vi "OP600ZP_FDT_V2.vi"(8 "errin":errorcluster, 9 "Tusine":dbl) -> (0 "errout":errorcluster, 2 "Log":string, 3 "is OK?":bool, 4 "ToBDD":T1)   [LabVIEW 2020]
uses:
  <userlib>/PCAN Basic/Controls/Channel.ctl
  VG/Ubatt.vi
  VG/PackType.vi
  VG/IS30%.vi
  OP600ZP_VGConf.vi
  <userlib>/PCAN Basic/PCANBasic.lvlib
panel:
  out "PASS/FAIL?":string
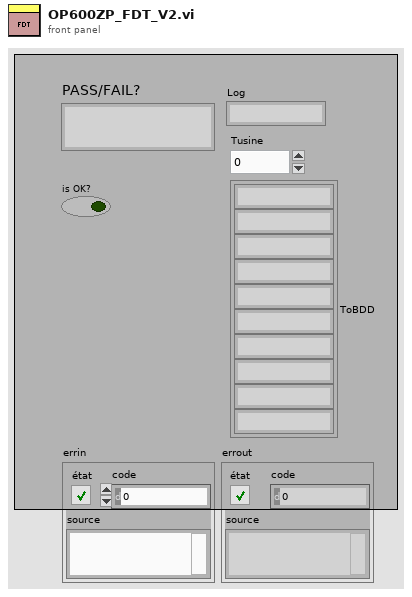
[diagram p1: front panel]
types:
  T1 = cluster{string, string, string, string, string, string, string, string, string, string}
  T2 = typedef "PCANBasic.lvlib/Channel.ctl" = enum16{"PCAN_NONEBUS", "not used1", "not used2", "not used3", "not used4", "not used5", "not used6", "not used7", "not used8", "not used9", "not used10", "not used11", "not used12", "not used13", "not used14", "not used15", "not used16", "not used17", "not used18", "not used19", "not used20", "not used21", "not used22", "not used23", "not used24", "not used25", "not used26", "not used27", "not used28", "not used29", "not used30", "not used31", "not used32", "PCAN_ISABUS1", "PCAN_ISABUS2", "PCAN_ISABUS3", "PCAN_ISABUS4", "PCAN_ISABUS5", "PCAN_ISABUS6", "PCAN_ISABUS7", "PCAN_ISABUS8", "not used41", "not used42", "not used43", "not used44", "not used45", "not used46", "not used47", "not used48", "PCAN_DNGBUS1", "not used50", "not used51", "not used52", "not used53", "not used54", "not used55", "not used56", "not used57", "not used58", "not used59", "not used60", "not used61", "not used62", "not used63", "not used64", "PCAN_PCIBUS1", "PCAN_PCIBUS2", "PCAN_PCIBUS3", "PCAN_PCIBUS4", "PCAN_PCIBUS5", "PCAN_PCIBUS6", "PCAN_PCIBUS7", "PCAN_PCIBUS8", "not used73", "not used74", "not used75", "not used76", "not used77", "not used78", "not used79", "not used80", "PCAN_USBBUS1", "PCAN_USBBUS2", "PCAN_USBBUS3", "PCAN_USBBUS4", "PCAN_USBBUS5", "PCAN_USBBUS6", "PCAN_USBBUS7", "PCAN_USBBUS8", "Not used89", "Not used90", "Not used91", "Not used92", "Not used93", "Not used94", "Not used95", "Not used96", "PCAN_PCCBUS1", "PCAN_PCCBUS2"}
  T3 = cluster{"F400 Battery Charge Type":string, "F400 Battery State Request":string, "F400 Ext Insulation Test Control":string, "F400 Int Insulation Test Control":string, "F400 Vehicle Speed":i32, "F400 Ambiant Temperature":i32, "F400 Charger Available Power":i32, "F400 Count":i32, "F106 Keep Active request":string, "F106 Battery State":string, "F106 Operating Status":string, "F106 Battery SOC":dbl, "F106 Battery SOH":dbl, "F106 Ext Insulation Test Status":string, "F106 Int Insulation Test Status":string, "F106 Power Distribution Status":string, "F106 Power Switch Off Delay":i32, "F106 Power Switch Off Request":string, "F106 Count":i32, "F101 Battery Voltage":u32, "F101 Battery Current":dbl, "F101 Max Charge Current":u32, "F101 Max Discharge Current":u32, "F101 Max Discharge Current Temp Limit":string, "F101 Max Discharge Current SOC Limit":string, "F101 Max Charge Current Temp Limit":string, "F101 Max Charge Current SOC Limit":string, "F101 Deliverable Energy":dbl, "F101 Count":u32, "F102 Cell Average Voltage":u32, "F102 Cell Min Voltage":u32, "F102 Cell Max Voltage":u32, "F103 Cell Average Temp":i32, "F103 Cell Min Temp":i32, "F102 Count":u32, "F103 SumOfInternalResistanceT":i32, "F100 Charge Voltage Setpoint":i32, "F100 Charge Current Setpoint":dbl, "F100 Equilization Status":bool, "F100 Charge Competed":bool, "F100 Count":i32, "F107 Outlet Water Temp Request":i32, "F107 Outlet Water Temp Status":i32, "F107 Flow Rate Request":i32, "F107 Inlet Water Temp":i32, "F107 Ambiant Temperature 2":i32, "F105 Max Power Charge Continuous":i32, "F105 Max Power Charge Long Prediction":i32, "F105 Max Power Charge Short Prediction":i32, "F105 Max Current Charge Continuous":i32, "F105 Max Current Charge Short Prediction":i32, "F105 Count ":i32, "F104 Max Power Discharge Continuous":i32, "F104 Max Power Discharge Long Prediction":i32, "F104 Max Power Discharge Short Prediction":i32, "F104 Max Current Discharge Continuous":i32, "F104 Max Current Discharge Short Prediction":i32, "F104 Count ":i32, "F103 Count":i32, "F103 Cell Max Temp":i32, "F103 Max Current Discharge Long Prediction":i32, "F103 Max Current Charge Long Prediction":i32, "F107 Count":i32, "F103 OCV":i32, "F109 DTC":i32}
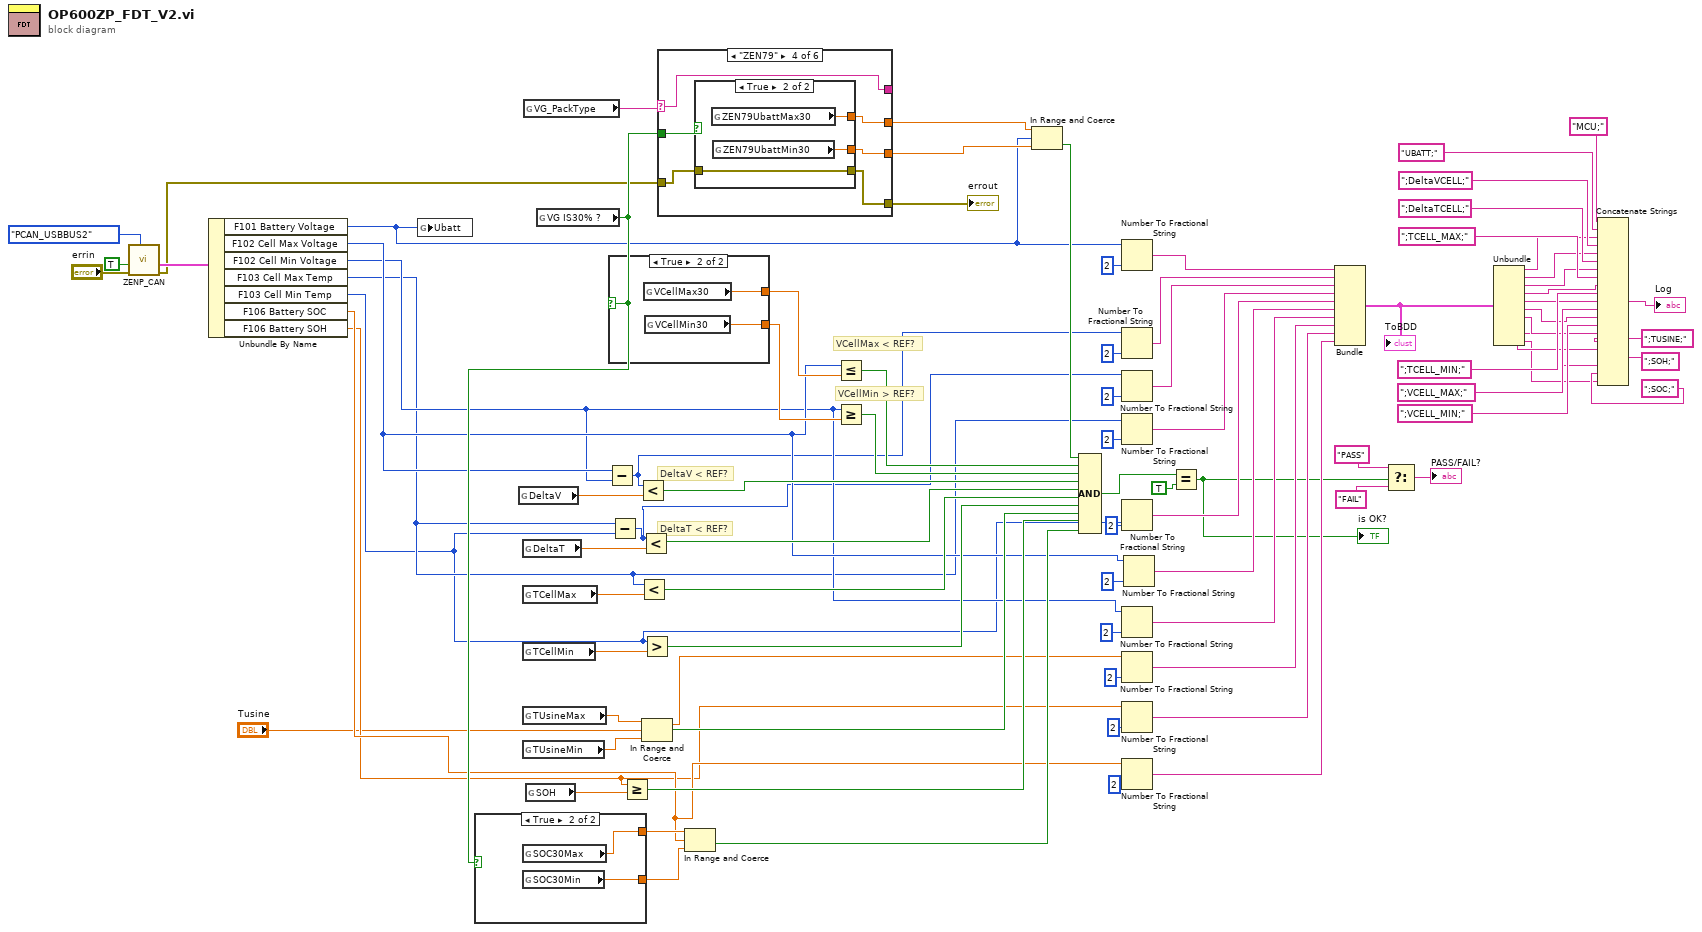
[diagram p0: block diagram]
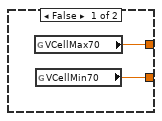
[diagram p2: hidden frame]
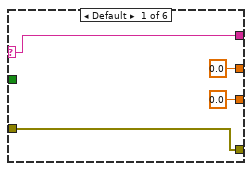
[diagram p3: hidden frame]
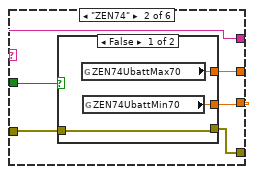
[diagram p4: hidden frame]
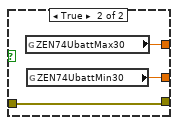
[diagram p5: hidden frame]
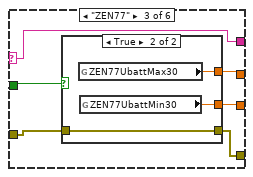
[diagram p6: hidden frame]
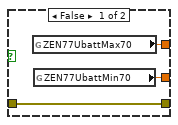
[diagram p7: hidden frame]
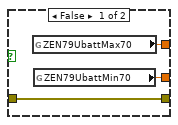
[diagram p8: hidden frame]
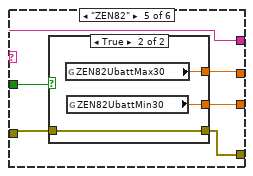
[diagram p9: hidden frame]
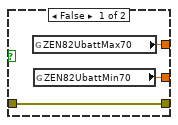
[diagram p10: hidden frame]
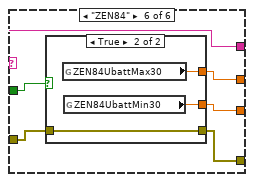
[diagram p11: hidden frame]
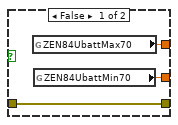
[diagram p12: hidden frame]
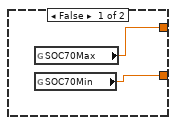
[diagram p13: hidden frame]
diagram:
  # "DeltaT < REF?"
  # "DeltaV < REF?"
  # "VCellMin > REF?"
  # "VCellMax < REF?"
  n1 = call <userlib>:"ZENP_CAN.vi"("Channel No Init"=Channel."PCAN_USBBUS2" ("Channel"), "errin"="errin", "Init?"=TRUE) -> ("errout"=w7:errorcluster, "data out"=w16:T3)  [unwired: 5 in, 1 out]
  n2 = Unbundle By Name(w16) -> ("F101 Battery Voltage"=w14:u32, "F102 Cell Max Voltage"=w13:u32, "F102 Cell Min Voltage"=w12:u32, "F103 Cell Max Temp"=w11:i32, "F103 Cell Min Temp"=w10:i32, "F106 Battery SOC"=w9:dbl, "F106 Battery SOH"=w8:dbl)
  n3 = global write "Ubatt.vi" "Ubatt"(w14) -> ()
  n4 = global read "OP600ZP_VGConf.vi" "DeltaV"() -> (w77:dbl)
  n5 = global read "OP600ZP_VGConf.vi" "DeltaT"() -> (w76:dbl)
  n6 = global read "OP600ZP_VGConf.vi" "TCellMax"() -> (w69:dbl)
  n7 = global read "OP600ZP_VGConf.vi" "TCellMin"() -> (w70:dbl)
  n8 = global read "OP600ZP_VGConf.vi" "TUsineMax"() -> (w64:dbl)
  n9 = global read "OP600ZP_VGConf.vi" "TUsineMin"() -> (w63:dbl)
  n10 = global read "PackType.vi" "VG_PackType"() -> (w91:string)
  n11 = global read "OP600ZP_VGConf.vi" "SOH"() -> (w29:dbl)
  n12 = global read "IS30%.vi" "VG IS30% ?"() -> (w32:bool)
  n13 = case shown="True" w32 {
    tunnel: [w93 w95] -> w31
    tunnel: [w92 w94] -> w30
    frame False {
      n14 = global read "OP600ZP_VGConf.vi" "SOC70Max"() -> (w93:dbl)
      n15 = global read "OP600ZP_VGConf.vi" "SOC70Min"() -> (w92:dbl)
    }
    frame True {
      n16 = global read "OP600ZP_VGConf.vi" "SOC30Max"() -> (w95:dbl)
      n17 = global read "OP600ZP_VGConf.vi" "SOC30Min"() -> (w94:dbl)
    }
  }
  n18 = Subtract(x=w13, y=w12) -> (x-y=w5:u32)
  n19 = case shown="True" w32 {
    tunnel: [w97 w99] -> w19
    tunnel: [w96 w98] -> w66
    frame False {
      n20 = global read "OP600ZP_VGConf.vi" "VCellMax70"() -> (w97:dbl)
      n21 = global read "OP600ZP_VGConf.vi" "VCellMin70"() -> (w96:dbl)
    }
    frame True {
      n22 = global read "OP600ZP_VGConf.vi" "VCellMax30"() -> (w99:dbl)
      n23 = global read "OP600ZP_VGConf.vi" "VCellMin30"() -> (w98:dbl)
    }
  }
  n24 = Subtract(x=w11, y=w10) -> (x-y=w4:i32)
  n25 = Greater Or Equal?(x=w8, y=w29) -> (x >= y?=w28:bool)
  n26 = Less?(x=w5, y=w77) -> (x < y?=w74:bool)
  n27 = Less?(x=w11, y=w69) -> (x < y?=w68:bool)
  n28 = Less?(x=w4, y=w76) -> (x < y?=w75:bool)
  n29 = Greater?(x=w10, y=w70) -> (0:w67:bool)
  n30 = In Range and Coerce(upper limit=w64, x="Tusine", lower limit=w63) -> (coerced(x)=w20:dbl, In Range?=w62:bool)
  n31 = case shown="\"ZEN79\"" w91 {
    selector: w91 -> [w103 w106 w118 w130 w142 w154]
    tunnel: [0.0 ("ZEN84UbattMax30") w109 w121 w133 w145 w157] -> w78
    tunnel: [0.0 ("ZEN84UbattMin30") w108 w120 w132 w144 w156] -> w79
    tunnel: w32 -> [_ w107 w119 w131 w143 w155]
    tunnel: [w103 w106 w118 w130 w142 w154] -> _
    tunnel: w7 -> [w102 w105 w117 w129 w141 w153]
    tunnel: [w102 w104 w116 w128 w140 w152] -> w90
    frame Default {
    }
    frame "ZEN74" {
      n32 = case shown="False" w107 {
        tunnel: [w112 w115] -> w109
        tunnel: [w111 w114] -> w108
        tunnel: [w110 w113] -> w104
        tunnel: w105 -> [w110 w113]
        frame False {
          n33 = global read "OP600ZP_VGConf.vi" "ZEN74UbattMax70"() -> (w112:dbl)
          n34 = global read "OP600ZP_VGConf.vi" "ZEN74UbattMin70"() -> (w111:dbl)
        }
        frame True {
          n35 = global read "OP600ZP_VGConf.vi" "ZEN74UbattMax30"() -> (w115:dbl)
          n36 = global read "OP600ZP_VGConf.vi" "ZEN74UbattMin30"() -> (w114:dbl)
        }
      }
    }
    frame "ZEN77" {
      n37 = case shown="True" w119 {
        tunnel: [w124 w127] -> w121
        tunnel: [w123 w126] -> w120
        tunnel: w117 -> [w122 w125]
        tunnel: [w122 w125] -> w116
        frame False {
          n38 = global read "OP600ZP_VGConf.vi" "ZEN77UbattMax70"() -> (w124:dbl)
          n39 = global read "OP600ZP_VGConf.vi" "ZEN77UbattMin70"() -> (w123:dbl)
        }
        frame True {
          n40 = global read "OP600ZP_VGConf.vi" "ZEN77UbattMax30"() -> (w127:dbl)
          n41 = global read "OP600ZP_VGConf.vi" "ZEN77UbattMin30"() -> (w126:dbl)
        }
      }
    }
    frame "ZEN79" {
      n42 = case shown="True" w131 {
        tunnel: [w136 w139] -> w133
        tunnel: [w135 w138] -> w132
        tunnel: w129 -> [w134 w137]
        tunnel: [w134 w137] -> w128
        frame False {
          n43 = global read "OP600ZP_VGConf.vi" "ZEN79UbattMax70"() -> (w136:dbl)
          n44 = global read "OP600ZP_VGConf.vi" "ZEN79UbattMin70"() -> (w135:dbl)
        }
        frame True {
          n45 = global read "OP600ZP_VGConf.vi" "ZEN79UbattMax30"() -> (w139:dbl)
          n46 = global read "OP600ZP_VGConf.vi" "ZEN79UbattMin30"() -> (w138:dbl)
        }
      }
    }
    frame "ZEN82" {
      n47 = case shown="True" w143 {
        tunnel: [w148 w151] -> w145
        tunnel: [w147 w150] -> w144
        tunnel: w141 -> [w146 w149]
        tunnel: [w146 w149] -> w140
        frame False {
          n48 = global read "OP600ZP_VGConf.vi" "ZEN82UbattMax70"() -> (w148:dbl)
          n49 = global read "OP600ZP_VGConf.vi" "ZEN82UbattMin70"() -> (w147:dbl)
        }
        frame True {
          n50 = global read "OP600ZP_VGConf.vi" "ZEN82UbattMax30"() -> (w151:dbl)
          n51 = global read "OP600ZP_VGConf.vi" "ZEN82UbattMin30"() -> (w150:dbl)
        }
      }
    }
    frame "ZEN84" {
      n52 = case shown="True" w155 {
        tunnel: [w160 w163] -> w157
        tunnel: [w159 w162] -> w156
        tunnel: w153 -> [w158 w161]
        tunnel: [w158 w161] -> w152
        frame False {
          n53 = global read "OP600ZP_VGConf.vi" "ZEN84UbattMax70"() -> (w160:dbl)
          n54 = global read "OP600ZP_VGConf.vi" "ZEN84UbattMin70"() -> (w159:dbl)
        }
        frame True {
          n55 = global read "OP600ZP_VGConf.vi" "ZEN84UbattMax30"() -> (w163:dbl)
          n56 = global read "OP600ZP_VGConf.vi" "ZEN84UbattMin30"() -> (w162:dbl)
        }
      }
    }
  }
  "errout" <- w90
  n57 = In Range and Coerce(upper limit=w31, x=w9, lower limit=w30) -> (In Range?=w27:bool)  [unwired: 1 out]
  n58 = Less Or Equal?(x=w13, y=w19) -> (x <= y?=w72:bool)
  n59 = Greater Or Equal?(x=w12, y=w66) -> (x >= y?=w73:bool)
  n60 = In Range and Coerce(upper limit=w78, x=w14, lower limit=w79) -> (In Range?=w71:bool)  [unwired: 1 out]
  n61 = Compound Arithmetic op=AND ("Opérateur arithmétique")(w71, w72, w73, w74, w75, w68, w67, w62, w28, w27) -> (w84:bool)
  n62 = Number To Fractional String(number=w14, precision (6)=i16 2 ("précision (6)")) -> (F-format string=w89:string)  [unwired: 2 in]
  n63 = Number To Fractional String(number=w5, precision (6)=i16 2 ("précision (6)")) -> (F-format string=w88:string)  [unwired: 2 in]
  n64 = Number To Fractional String(number=w4, precision (6)=i16 2 ("précision (6)")) -> (F-format string=w87:string)  [unwired: 2 in]
  n65 = Number To Fractional String(number=w11, precision (6)=i16 2 ("précision (6)")) -> (F-format string=w86:string)  [unwired: 2 in]
  n66 = Number To Fractional String(number=w10, precision (6)=i16 2 ("précision (6)")) -> (F-format string=w85:string)  [unwired: 2 in]
  n67 = Number To Fractional String(number=w12, precision (6)=i16 2 ("précision (6)")) -> (F-format string=w65:string)  [unwired: 2 in]
  n68 = Number To Fractional String(number=w20, precision (6)=i16 2 ("précision (6)")) -> (F-format string=w61:string)  [unwired: 2 in]
  n69 = Number To Fractional String(number=w8, precision (6)=i16 2 ("précision (6)")) -> (F-format string=w26:string)  [unwired: 2 in]
  n70 = Number To Fractional String(number=w9, precision (6)=i16 2 ("précision (6)")) -> (F-format string=w25:string)  [unwired: 2 in]
  n71 = Number To Fractional String(number=w13, precision (6)=i16 2 ("précision (6)")) -> (F-format string=w18:string)  [unwired: 2 in]
  n72 = Equal?(x=w84, y=TRUE) -> (x = y?=w3:bool)
  "is OK?" <- w3
  n73 = Bundle(w89, w88, w87, w86, w85, w18, w65, w61, w26, w25) -> (w36:T1)  [unwired: 1 in]
  "ToBDD" <- w36
  n74 = Select ("Sélectionner")(t="PASS", s=w3, f="FAIL") -> (s? t:f=→"PASS/FAIL?":string)
  n75 = Unbundle(w36) -> (w45:string, w44:string, w43:string, w42:string, w41:string, w40:string, w39:string, w37:string, w23:string, w21:string)
  n76 = Concatenate Strings("MCU;" ("chaîne"), "UBATT;", w45, ";DeltaVCELL;", w44, ";DeltaTCELL;", w43, ";TCELL_MAX;", w42, ";TCELL_MIN;", w41, ";VCELL_MAX;", w40, ";VCELL_MIN;", w39, ";TUSINE;" ("chaîne"), w37, ";SOH;" ("chaîne"), w23, ";SOC;" ("chaîne"), w21) -> (→"Log":string)
